vi "AppenderConfigDTOFromNative.vi"(8 "error in (no error)":errorcluster, 11 "AppenderConfig":T1={"id"="", "threshold"=enum."INFO", "filter"={"mode"=enum."Mirror", "levelMin"=enum."INFO", "levelMax"=enum."INFO", "tagPrefix"=""}, "queueBound"=0, "dropPolicy"=enum."DropOldest"}) -> (0 "error out":errorcluster, 3 "AppenderConfigDTO":T6={"id"="", "threshold"="INFO", "filter"={"mode"="Mirror", "levelMin"="INFO", "levelMax"="INFO", "tagPrefix"=""}, "queueBound"=0, "dropPolicy"="DropOldest"})   [LabVIEW 2026, in "Lumberjack.lvlib"]
uses:
  Lumberjack.lvlib
  TypeDefs/ConfigDTO/AppenderConfigDTO.ctl
  TypeDefs/ConfigDTO/FilterDTO.ctl
  TypeDefs/AppenderConfig.ctl
  TypeDefs/Severity.ctl
  TypeDefs/Filter.ctl
  TypeDefs/FilterMode.ctl
  TypeDefs/DropPolicy.ctl
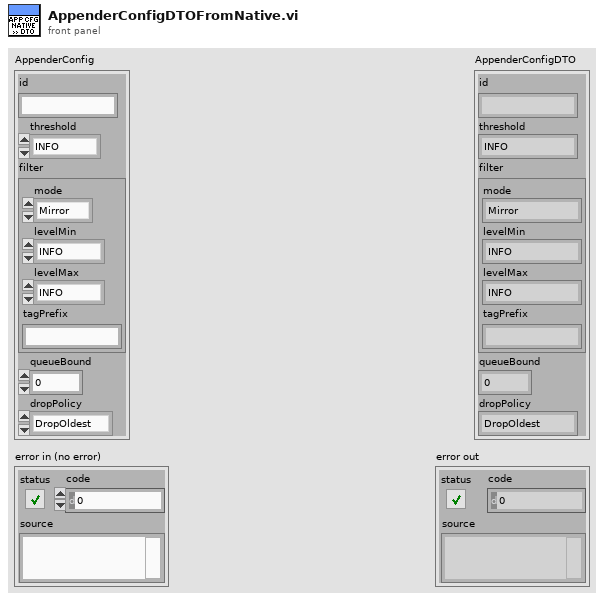
[diagram p1: front panel]
types:
  T1 = typedef "Lumberjack.lvlib/AppenderConfig.ctl" = cluster{"id":string, "threshold":T2, "filter":T3, "queueBound":i32, "dropPolicy":T5}
  T2 = typedef "Lumberjack.lvlib/Severity.ctl" = enum16{"OFF", "FATAL", "ERROR", "WARN", "INFO", "DEBUG", "TRACE", "ALL"}
  T3 = typedef "Lumberjack.lvlib/Filter.ctl" = cluster{"mode":T4, "levelMin":T2, "levelMax":T2, "tagPrefix":string}
  T4 = typedef "Lumberjack.lvlib/FilterMode.ctl" = enum16{"Mirror", "Routed"}
  T5 = typedef "Lumberjack.lvlib/DropPolicy.ctl" = enum16{"DropOldest", "DropNewest", "LevelAware"}
  T6 = typedef "Lumberjack.lvlib/AppenderConfigDTO.ctl" = cluster{"id":string, "threshold":string, "filter":T7, "queueBound":i32, "dropPolicy":string}
  T7 = typedef "Lumberjack.lvlib/FilterDTO.ctl" = cluster{"mode":string, "levelMin":string, "levelMax":string, "tagPrefix":string}
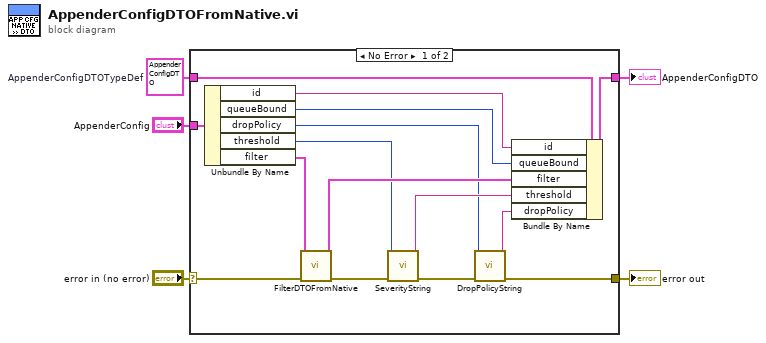
[diagram p0: block diagram]
diagram:
  w4 = T6 {"id"="", "threshold"="INFO", "filter"={"mode"="Mirror", "levelMin"="INFO", "levelMax"="INFO", "tagPrefix"=""}, "queueBound"=0, "dropPolicy"="DropOldest"}  # AppenderConfigDTOTypeDef
  n1 = case shown="No Error" "error in (no error)" {
    selector: "error in (no error)" -> [w20 w22]
    tunnel: [w17 w22] -> w2
    tunnel: "AppenderConfig" -> [w15 _]
    tunnel: w4 -> [w14 w21]
    tunnel: [w16 w21] -> w1
    frame No Error {
      n2 = Unbundle By Name(w15) -> ("id"=w13:string, "queueBound"=w12:i32, "dropPolicy"=w7:T5, "threshold"=w9:T2, "filter"=w11:T3)
      n3 = call "FilterDTOFromNative.vi"("error in (no error)"=w20, "Filter"=w11) -> ("error out"=w19:errorcluster, "FilterDTO"=w10:T7)  [unwired: 8 in]
      n4 = call "SeverityString.vi"("error in (no error)"=w19, "Severity"=w9) -> ("error out"=w18:errorcluster, "SeverityString"=w8:string)  [unwired: 8 in]
      n5 = call "DropPolicyString.vi"("error in (no error)"=w18, "DropPolicy"=w7) -> ("error out"=w17:errorcluster, "FilterModeString"=w6:string)  [unwired: 8 in]
      n6 = Bundle By Name(cluster=w14, "id"=w13, "queueBound"=w12, "filter"=w10, "threshold"=w8, "dropPolicy"=w6) -> (w16:T6)
    }
    frame Error {
    }
  }
  "AppenderConfigDTO" <- w1
  "error out" <- w2
